vi "getOptSetting.vi"(6 "addr/port":cluster{"address":string, "port":i32}={"address"="127.0.0.1", "port"=31415}, 8 "error in (no error)":errorcluster) -> (0 "error out":errorcluster, 3 "setting":dbl)   [LabVIEW 2015]
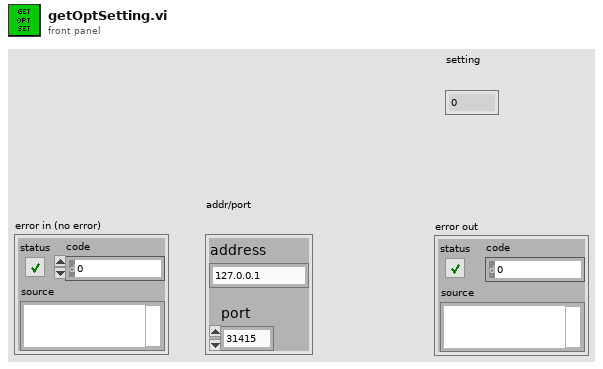
[diagram p1: front panel]
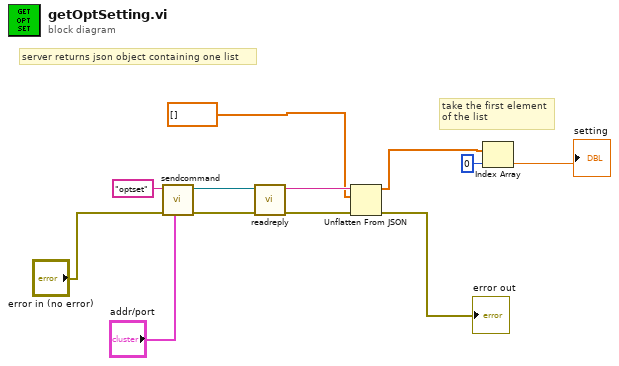
[diagram p0: block diagram]
diagram:
  # "take the first element\nof the list"
  # "server returns json object containing one list"
  n1 = call "sendcommand.vi"("addr/port"="addr/port", "error in (no error)"="error in (no error)", "command"="optset") -> ("error out"=w8:errorcluster, "connection ID out"=w9:refnum<k5>)  [unwired: 6 in, 1 out]
  n2 = call "readreply.vi"("error in (no error)"=w8, "connection ID"=w9) -> ("error out"=w7:errorcluster, "data out"=w5:string)  [unwired: 8 in]
  n3 = Unflatten From JSON(JSON string=w5, type and defaults=dbl[] [] ("Array"), error in (no error)=w7) -> (value=w1:dbl[], error out=→"error out":errorcluster)  [unwired: 4 in]
  n4 = Index Array(array=w1, index=0) -> (element=→"setting":dbl)
